vi "Write GIF File (Animated) Example.vi"(8 "error in (no error)":errorcluster) -> (0 "error out":errorcluster)   [LabVIEW 2009]
panel:
  out "pre check":bool
  out "post check":bool
  out "post check":bool
  out "Array 2":u32[][][](array[colorbox])
  in  "Array":u32[][][](array[colorbox])=array75x36x36[97200 elements]
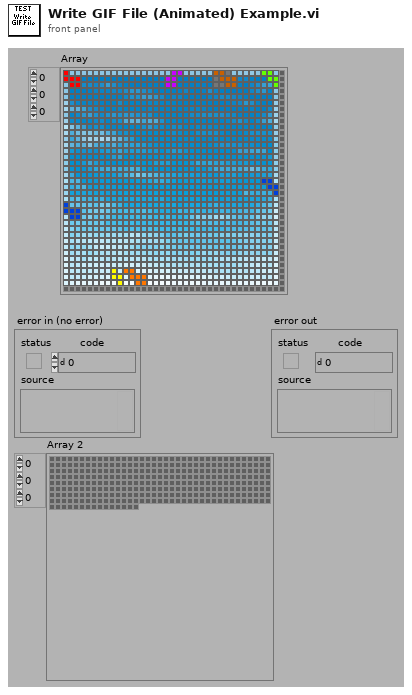
[diagram p1: front panel]
types:
  T1 = typedef "imagedata.ctl" = cluster{"image type":i32, "image depth":i32, "image":u8[], "mask":u8[], "colors":u32[], "Rectangle":cluster{"left":i16, "top":i16, "right":i16, "bottom":i16}}
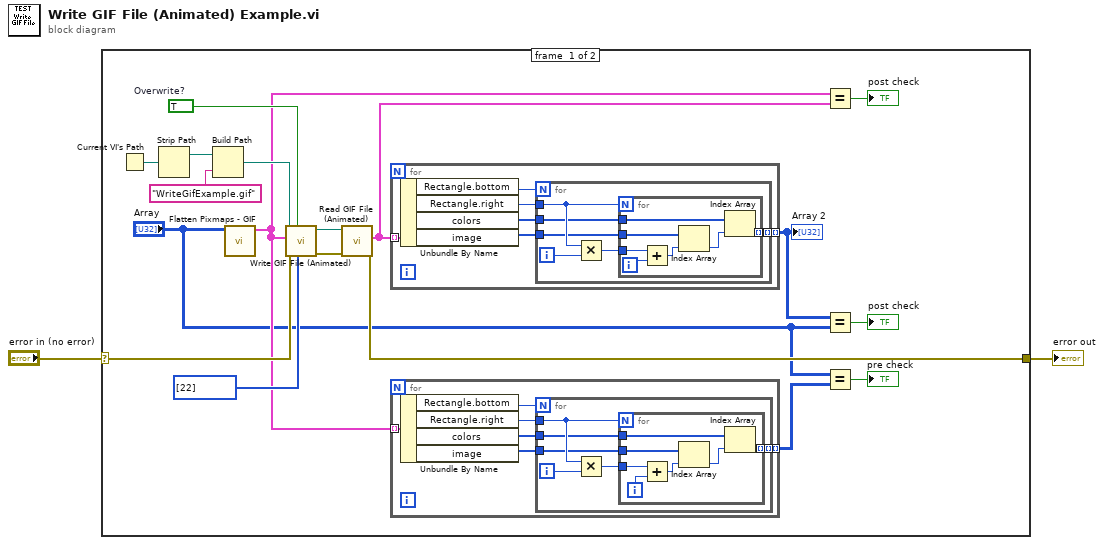
[diagram p0: block diagram]
diagram:
  n1 = case shown="No Error" "error in (no error)" {
    selector: "error in (no error)" -> [w20 w59]
    tunnel: [w12 w59] -> w1
    frame #0 {
      w18 = TRUE  # Overwrite?
      n2 = Current VI's Path() -> (path=w15:path)
      n3 = Strip Path(path=w15) -> (stripped path=w14:path)  [unwired: 1 out]
      n4 = Build Path(base path=w14, name or relative path="WriteGifExample.gif") -> (appended path=w17:path)
      n5 = call "Flatten Pixmaps - GIF.vi"("PixelTable"="Array") -> ("Images"=w6:T1[])  [unwired: 10 in]
      n6 = call "Write GIF File (Animated).vi"("delay (ms)"=i32[] [22], "overwrite? (false)"=w18, "error in (no error)"=w20, "images data"=w6, "path to GIF file"=w17) -> ("error out"=w16:errorcluster, "path"=w13:path)  [unwired: 5 in]
      n7 = call "Read GIF File (Animated).vi"("error in (no error)"=w16, "path to GIF file"=w13) -> ("error out"=w12:errorcluster, "images data"=w8:T1[])  [unwired: 5 in, 3 out]
      n8 = for {
        tunnel: w8 -> [w45] mode=indexing
        tunnel: [w40] -> w10 mode=indexing
        n9 = Unbundle By Name(w45) -> ("Rectangle.bottom"=w44:i16, "Rectangle.right"=w43:i16, "colors"=w42:u32[], "image"=w41:u8[])
        n10 = for {
          N: w44 -> [_]
          tunnel: w43 -> [w50]
          tunnel: w42 -> [w49]
          tunnel: w41 -> [w48]
          tunnel: [w46] -> w40 mode=indexing
          i -> [w51]
          n11 = Multiply(x=w50, y=w51) -> (x*y=w47:i32)
          n12 = for {
            N: w50 -> [_]
            tunnel: w49 -> [w58]
            tunnel: w48 -> [w57]
            tunnel: w47 -> [w56]
            tunnel: [w52] -> w46 mode=indexing
            i -> [w55]
            n13 = Add(x=w56, y=w55) -> (x+y=w54:i32)
            n14 = Index Array(array=w57, index=w54) -> (element=w53:u8)
            n15 = Index Array(array=w58, index=w53) -> (element=w52:u32)
          }
        }
      }
      "Array 2" <- w10
      n16 = for {
        tunnel: w6 -> [w26] mode=indexing
        tunnel: [w21] -> w4 mode=indexing
        n17 = Unbundle By Name(w26) -> ("Rectangle.bottom"=w25:i16, "Rectangle.right"=w24:i16, "colors"=w23:u32[], "image"=w22:u8[])
        n18 = for {
          N: w25 -> [_]
          tunnel: w24 -> [w31]
          tunnel: w23 -> [w30]
          tunnel: w22 -> [w29]
          tunnel: [w27] -> w21 mode=indexing
          i -> [w32]
          n19 = Multiply(x=w31, y=w32) -> (x*y=w28:i32)
          n20 = for {
            N: w31 -> [_]
            tunnel: w30 -> [w39]
            tunnel: w29 -> [w38]
            tunnel: w28 -> [w37]
            tunnel: [w33] -> w27 mode=indexing
            i -> [w36]
            n21 = Add(x=w37, y=w36) -> (x+y=w35:i32)
            n22 = Index Array(array=w38, index=w35) -> (element=w34:u8)
            n23 = Index Array(array=w39, index=w34) -> (element=w33:u32)
          }
        }
      }
      n24 = Equal?(x=w6, y=w8) -> (x = y?=→"post check":bool)
      n25 = Equal?(x=w10, y="Array") -> (x = y?=→"post check":bool)
      n26 = Equal?(x="Array", y=w4) -> (x = y?=→"pre check":bool)
    }
    frame #1 {
    }
  }
  "error out" <- w1
